vi "Find Workspace.vi"(8 "Error In":errorcluster, 9 "Type of Hexaboard":T1, 10 "Control In":T3={"I-O.lvclass"=refnum, "Gantry"=refnum, "Dispenser"="COM1"}, 11 "Carrier Tray in":refnum<class "Assembly Tray.lvclass">) -> (0 "Error Out":errorcluster, 1 "Workspace":T2, 2 "Control Out":T3={"I-O.lvclass"=refnum, "Gantry"=refnum, "Dispenser"="COM1"}, 3 "Carrier Tray Out":refnum<class "Assembly Tray.lvclass">)   [LabVIEW 2021, in "Assembly Tray.lvclass"]
uses:
  Assembly Tray.lvclass
  C:/Users/hep/Documents/UCSB-CMU-GantryCode/UCSB-Gantry-HEP-main (3)/UCSB-Gantry-HEP-main/Classes/Workspace/Fixture.lvclass
  Controller/Controllers.ctl
  Controller/I-O/I-O.lvclass
  C:/Program Files (x86)/Aerotech/A3200/LabVIEW/2010/Bin/Aerotech.A3200.dll
  Program Files (x86)/Aerotech/A3200/LabVIEW/2010/Bin/Aerotech.A3200.dll
  Workspace.ctl
  Routine/TypeOfHexaboard.ctl
  Fixture.lvclass/Fixture.ctl
  Assembly Tray.lvclass/Assembly Tray.ctl
  Read Fixture ID.vi
  Read Position.vi
  Fixture.lvclass
  Controller/Controller.lvclass
  Routine/Routine.lvclass
panel:
  out "XYZTheta Centers":dbl[][](array[numeric])
  in  "output cluster 2":T2
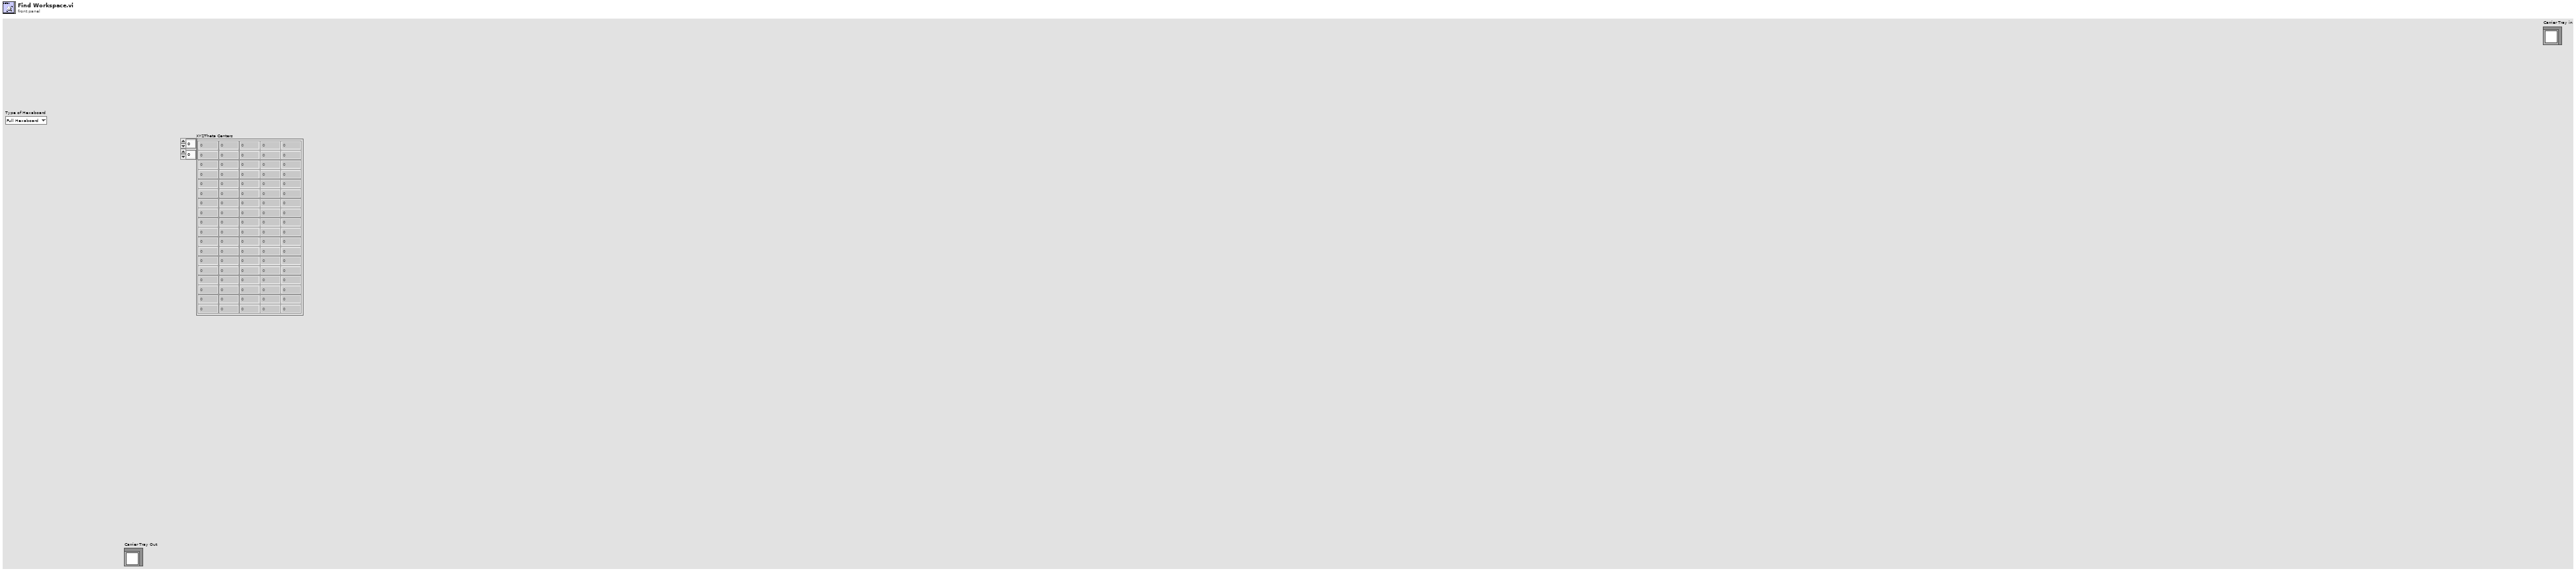
[diagram p1: front panel]
types:
  T1 = typedef "Routine.lvclass/TypeOfHexaboard.ctl" = enum16{"Full Hexaboard", "Right Partial PCB", "Right Partial Sensor", "Al Dummy Right Partial Sensor"}
  T2 = typedef "Fixture.lvclass/Workspace.ctl" = cluster{"XYZTheta":dbl[], "Workspace Valve":i32, "Workspace Sensor":i32}
  T3 = typedef "Controller.lvclass/Controllers.ctl" = cluster{"I-O.lvclass":refnum<class "I-O.lvclass">, "Gantry":refnum<k24>, "Dispenser":refnum<visa-resource-name>}
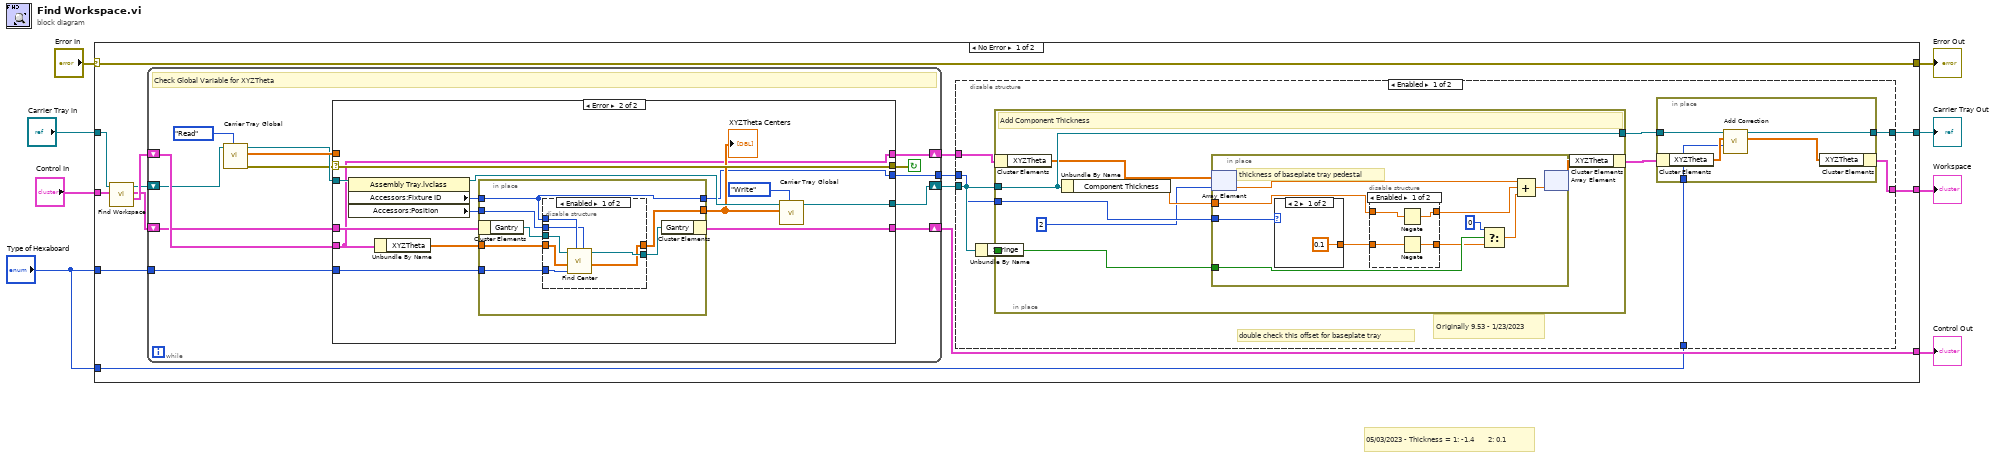
[diagram p0: block diagram]
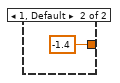
[diagram p2: hidden frame]
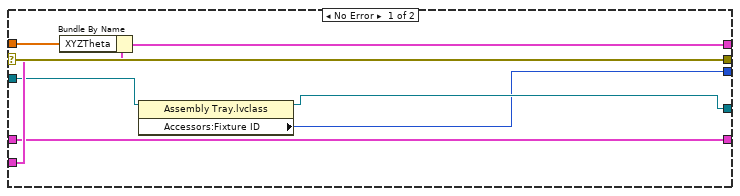
[diagram p5: hidden frame]
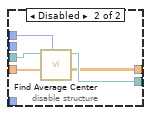
[diagram p6: hidden frame]
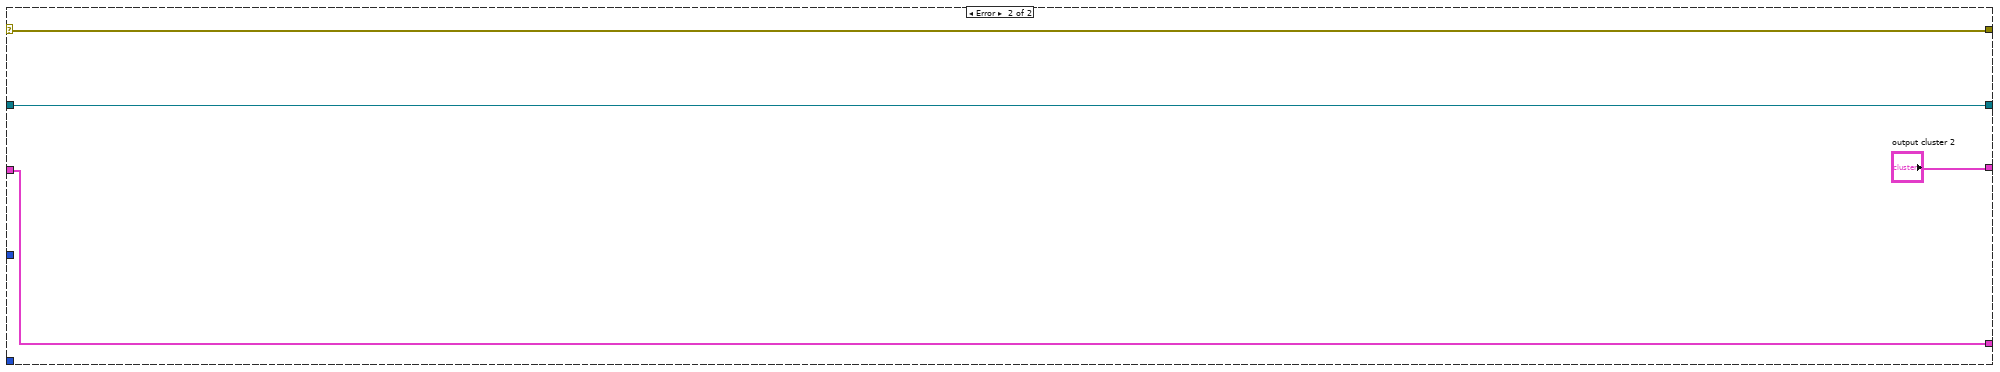
[diagram p7: hidden frame]
diagram:
  # "05/03/2023 - Thickness = 1: -1.4       2: 0.1"
  n1 = case shown="No Error" "Error In" {
    selector: "Error In" -> [w22 w120]
    tunnel: [w22 w120] -> w7
    tunnel: "Control In" -> [w21 w121]
    tunnel: [w17 w121] -> w5
    tunnel: "Carrier Tray in" -> [w20 w118]
    tunnel: [w18 "output cluster 2"] -> w3
    tunnel: [w19 w118] -> w2
    tunnel: "Type of Hexaboard" -> [w11 _]
    tunnel: "Type of Hexaboard" -> [w9 _]
    frame No Error {
      n2 = call-parent "Find Workspace.vi"("Control In"=w21, "Workspace In"=w20) -> (1:"Workspace Out"=w16:T2, "Control Out"=w15:T3, 3:"Workspace Out"=w12:refnum<class "Assembly Tray.lvclass">)  [unwired: 6 in, 1 out]
      n3 = while {
        shift-right: [w69] -> w14
        shift-left: w12 -> [w67]
        shift-right: [w71] -> w17
        shift-left: w15 -> [w72]
        shift-right: [w68] -> w13
        shift-left: w16 -> [w73]
        tunnel: w11 -> [w65]
        tunnel: [w64] -> w10
        stop <- w75 continue-if-true
        # "Check Global Variable for XYZTheta"
        n4 = call "Carrier Tray Global.vi"("Action"=enum16{"Initialize", "Read", "Write"}."Read", "Carrier Tray.lvclass"=w67) -> ("error out"=w66:errorcluster, "XYZTheta out"=w74:dbl[], "Carrier Tray.lvclass 2"=w70:refnum<class "Assembly Tray.lvclass">)  [unwired: 7 in]
        n5 = case shown="Error" w66 {
          selector: w66 -> [w84 w98]
          tunnel: [w84 w98] -> w75
          tunnel: w74 -> [w83 _]
          tunnel: [w82 w88] -> w68
          tunnel: w73 -> [w81 w88]
          tunnel: w72 -> [w80 w92]
          tunnel: [w80 w91] -> w71
          tunnel: w70 -> [w79 w95]
          tunnel: [w78 w97] -> w69
          tunnel: w65 -> [_ w87]
          tunnel: [w77 w85] -> w64
          frame No Error {
            n6 = Bundle By Name(cluster=w81, "XYZTheta"=w83) -> (w82:T2)
            n7 = property class="Assembly Tray.lvclass"(reference=w79) -> (reference out=w78:refnum<class "Assembly Tray.lvclass">, "Accessors:Fixture ID"=w77:i32)  [unwired: 1 in, 1 out]
          }
          frame Error {
            n8 = property class="Assembly Tray.lvclass"(reference=w95) -> (reference out=w94:refnum<class "Assembly Tray.lvclass">, "Accessors:Fixture ID"=w93:i32, "Accessors:Position"=w86:i32)  [unwired: 1 in, 1 out]
            n9 = Unbundle By Name(w88) -> ("XYZTheta"=w90:dbl[])
            n10 = in-place {
              in-place-border: w93 -> [w99]
              in-place-border: w90 -> [w103]
              in-place-border: [w102] -> w89
              in-place-border: w87 -> [w101]
              in-place-border: w86 -> [w100]
              in-place-border: [w99] -> w85
              n11 = in-place-cluster #1(w92) -> ("Gantry"=w105:refnum<k24>)
              n12 = disable-structure shown="Enabled" {
                disable-tunnel: w99 -> [w112 w113]
                disable-tunnel: w105 -> [w111 w117]
                disable-tunnel: [w110 w116] -> w104
                disable-tunnel: w103 -> [w109 w115]
                disable-tunnel: [w108 w114] -> w102
                disable-tunnel: w101 -> [w107 _]
                disable-tunnel: w100 -> [w106 _]
                frame Enabled {
                  n13 = call "Find Center.vi"("Position"=w106, "Tray Number"=w112, "Type of Hexaboard"=w107, "XYZTheta"=w109, "Gantry In"=w111) -> ("XYZTheta Centers"=w108:dbl[][], "Gantry Out"=w110:refnum<k24>)  [unwired: 5 in]
                }
                frame Disabled {
                  n14 = call "Find Average Center.vi"("Tray Number"=w113, "XYZTheta"=w115, "Gantry In"=w117) -> ("XYZTheta Centers"=w114:dbl[][], "Gantry Out"=w116:refnum<k24>)  [unwired: 7 in]
                }
              }
              n15 = in-place-cluster #1("Gantry"=w104) -> (w91:T3)
            }
            "XYZTheta Centers" <- w89
            n16 = call "Carrier Tray Global.vi"("Action"=enum16{"Initialize", "Read", "Write"}."Write", "XYZTheta in"=w89, "Carrier Tray.lvclass"=w94) -> ("Carrier Tray.lvclass 2"=w97:refnum<class "Assembly Tray.lvclass">)  [unwired: 6 in, 2 out]
          }
        }
      }
      n17 = disable-structure shown="Enabled" {
        disable-tunnel: [w31 w62] -> w19
        disable-tunnel: [w30 w63] -> w18
        disable-tunnel: w14 -> [w29 w62]
        disable-tunnel: w13 -> [w28 w63]
        disable-tunnel: w10 -> [w24 _]
        disable-tunnel: w9 -> [w23 _]
        frame Enabled {
          # "Originally 9.53 - 1/23/2023"
          # "double check this offset for baseplate tray"
          n18 = Unbundle By Name(w29) -> ("Syringe"=w27:bool)
          n19 = in-place {
            in-place-border: w29 -> [w41]
            in-place-border: [w41] -> w26
            in-place-border: w27 -> [w40]
            in-place-border: w24 -> [w38]
            # "Add Component Thickness"
            n20 = in-place-cluster #2(w28) -> ("XYZTheta"=w39:dbl[])
            n21 = Unbundle By Name(w41) -> ("Component Thickness"=w42:dbl)
            n22 = in-place {
              in-place-border: w42 -> [w48]
              in-place-border: w40 -> [w52]
              in-place-border: w38 -> [w44]
              # "thickness of baseplate tray pedestal"
              n23 = in-place-array #3(w39, 2) -> (w49:dbl)
              n24 = case shown="2" w44 {
                tunnel: [0.1 -1.4] -> w46
                frame 2 {
                }
                frame 1, Default {
                }
              }
              n25 = disable-structure shown="Enabled" {
                disable-tunnel: w48 -> [w59 w61]
                disable-tunnel: [w58 w61] -> w47
                disable-tunnel: w46 -> [w57 w60]
                disable-tunnel: [w56 w60] -> w45
                frame Enabled {
                  n26 = Negate(x=w59) -> (-x=w58:dbl)
                  n27 = Negate(x=w57) -> (-x=w56:dbl)
                }
                frame Disabled {
                }
              }
              n28 = Select(t=0, s=w52, f=w45) -> (s? t:f=w50:dbl)
              n29 = Compound Arithmetic op=ADD(w49, w47, w50) -> (w53:dbl)
              n30 = in-place-array #3(w53) -> (w43:dbl[])  [unwired: 1 out]
            }
            n31 = in-place-cluster #2("XYZTheta"=w43) -> (w25:T2)
          }
          n32 = in-place {
            in-place-border: [w36] -> w31
            in-place-border: w26 -> [w35]
            in-place-border: w23 -> [w32]
            n33 = in-place-cluster #4(w25) -> ("XYZTheta"=w34:dbl[])
            n34 = call "Add Correction.vi"("Type of Hexaboard"=w32, "XYZTheta"=w34, "Carrier Tray in"=w35) -> ("XYZTheta Out"=w33:dbl[], "Carrier Tray out"=w36:refnum<class "Assembly Tray.lvclass">)  [unwired: 6 in, 1 out]
            n35 = in-place-cluster #4("XYZTheta"=w33) -> (w30:T2)
          }
        }
        frame Disabled {
        }
      }
    }
    frame Error {
    }
  }
  "Error Out" <- w7
  "Control Out" <- w5
  "Workspace" <- w3
  "Carrier Tray Out" <- w2
